vi "niScope Fetch Error Chain.vi"(5 "dataType in":i32, 9 "error in":errorcluster) -> (8 "dataType":i32)   [LabVIEW 2013]
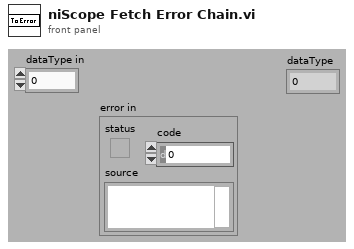
[diagram p1: front panel]
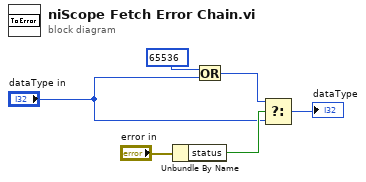
[diagram p0: block diagram]
diagram:
  n1 = Unbundle By Name("error in") -> ("status"=w3:bool)
  n2 = Or(x=65536, y="dataType in") -> (x .or. y?=w4:i32)
  n3 = Select(t=w4, s=w3, f="dataType in") -> (s? t:f=→"dataType":i32)
